vi "update_issue_cover_date.vi"(9 "issues in":i32, 10 "Cover Date":timestamp, 11 "issues 3":T1[](array[typedef])) -> (2 "issue":T1, 3 "issues out":T1[](array[typedef]))   [LabVIEW 2024]
uses:
  CV_RESTful_Library/typedefs/local_issue--cluster.ctl
  CV_RESTful_Library/typedefs/cv_issue.generic_credit--cluster.ctl
  CV_RESTful_Library/typedefs/cv_issue.associated_image--cluster.ctl
  CV_RESTful_Library/typedefs/cv_issue.person_credit--cluster.ctl
  CV_RESTful_Library/CV_RESTful_Lib.lvlib
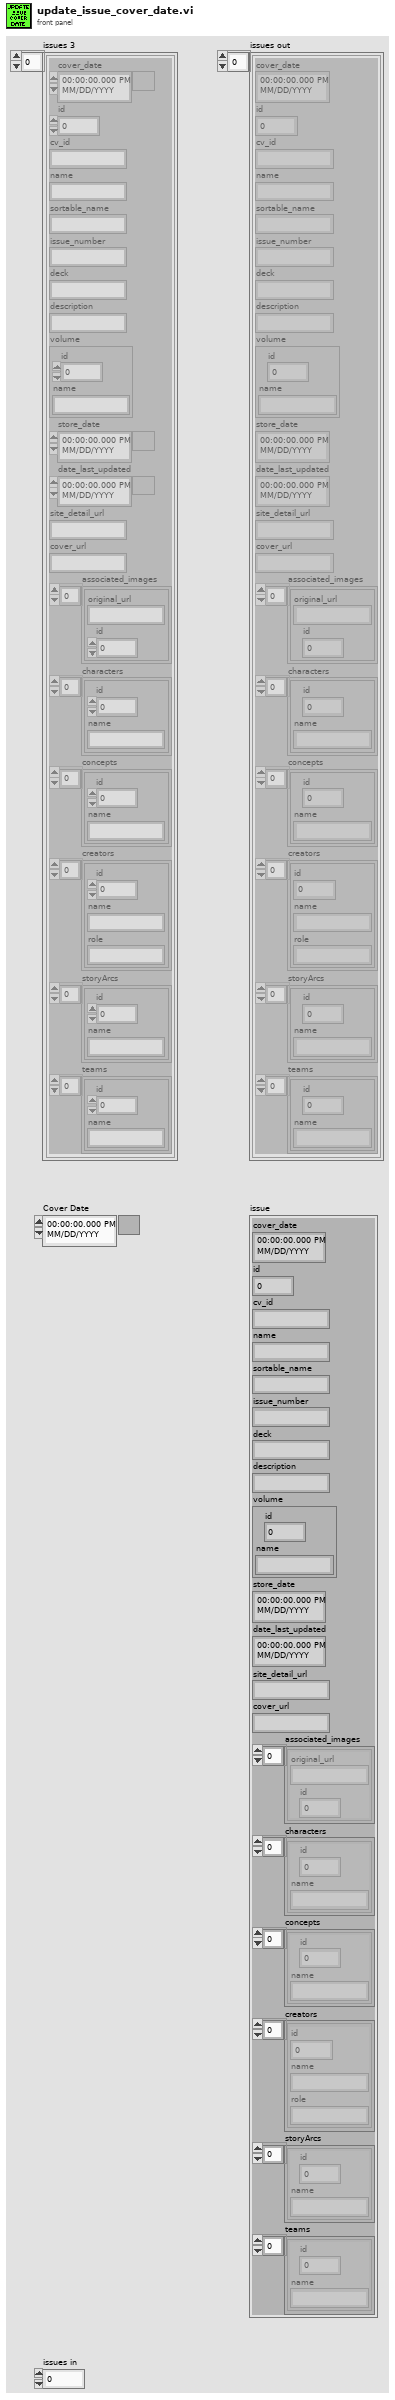
[diagram p1: front panel]
types:
  T1 = typedef "CV_RESTful_Lib.lvlib/local_issue--cluster.ctl" = cluster{"cover_date":timestamp, "id":i32, "cv_id":string, "name":string, "sortable_name":string, "issue_number":string, "deck":string, "description":string, "volume":T2, "store_date":timestamp, "date_last_updated":timestamp, "site_detail_url":string, "cover_url":string, "associated_images":T3[], "characters":T2[], "concepts":T2[], "creators":T4[], "storyArcs":T2[], "teams":T2[]}
  T2 = typedef "CV_RESTful_Lib.lvlib/cv_issue.generic_credit--cluster.ctl" = cluster{"id":i32, "name":string}
  T3 = typedef "CV_RESTful_Lib.lvlib/cv_issue.associated_image--cluster.ctl" = cluster{"original_url":string, "id":i32}
  T4 = typedef "CV_RESTful_Lib.lvlib/cv_issue.person_credit--cluster.ctl" = cluster{"id":i32, "name":string, "role":string}
  T5 = typedef "LVDateTimeRec.ctl" = cluster{"fractional second":dbl, "second":i32, "minute":i32, "hour":i32, "day of month":i32, "month":i32, "year":i32, "day of week":i32, "day of year":i32, "DST":i32}
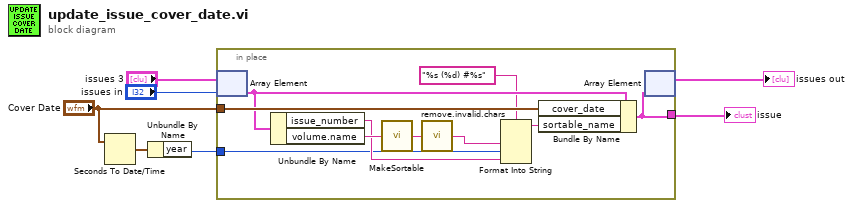
[diagram p0: block diagram]
diagram:
  n1 = Seconds To Date/Time(time stamp (now)="Cover Date") -> (date time rec=w5:T5)  [unwired: 1 in]
  n2 = Unbundle By Name(w5) -> ("year"=w7:i32)
  n3 = in-place {
    in-place-border: "Cover Date" -> [w17]
    in-place-border: [w16] -> w4
    in-place-border: w7 -> [w9]
    n4 = in-place-array #1("issues 3", "issues in") -> (w15:T1)
    n5 = Unbundle By Name(w15) -> ("issue_number"=w10:string, "volume.name"=w11:string)
    n6 = call "MakeSortable.vi"("string in"=w11) -> ("string out"=w13:string)
    n7 = call "remove.invalid.chars.vi"("string in"=w13) -> ("string out"=w12:string)
    n8 = Format Into String(format string="%s (%d) #%s", w12, w9, w10) -> (resulting string=w14:string)  [unwired: 2 in, 1 out]
    n9 = Bundle By Name(cluster=w15, "cover_date"=w17, "sortable_name"=w14) -> (w16:T1)
    n10 = in-place-array #1(w16) -> (→"issues out":T1[])  [unwired: 1 out]
  }
  "issue" <- w4
